vi "monitor_log_queue.vi"(6 "occurrence":refnum<k4>, 11 "File Log Provider in":refnum<data-value>) -> ()   [LabVIEW 2019, in "File Log Provider.lvclass"]
uses:
  File Log Provider.lvclass
  File Log Provider.lvclass/File Log Provider.ctl
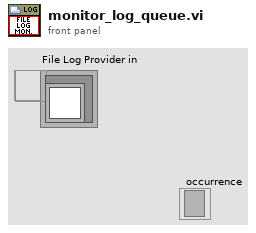
[diagram p1: front panel]
types:
  T1 = enum16{"open", "replace", "create", "open or create", "replace or create", "replace or create with confirmation"}
  T2 = typedef "Queue Log Provider.lvclass/log_message.ctl" = cluster{"Time Stamp":timestamp, "level":T3, "context":string, "message":string}
  T3 = typedef "Utility API.lvlib/Log Service.lvclass/level.ctl" = u16
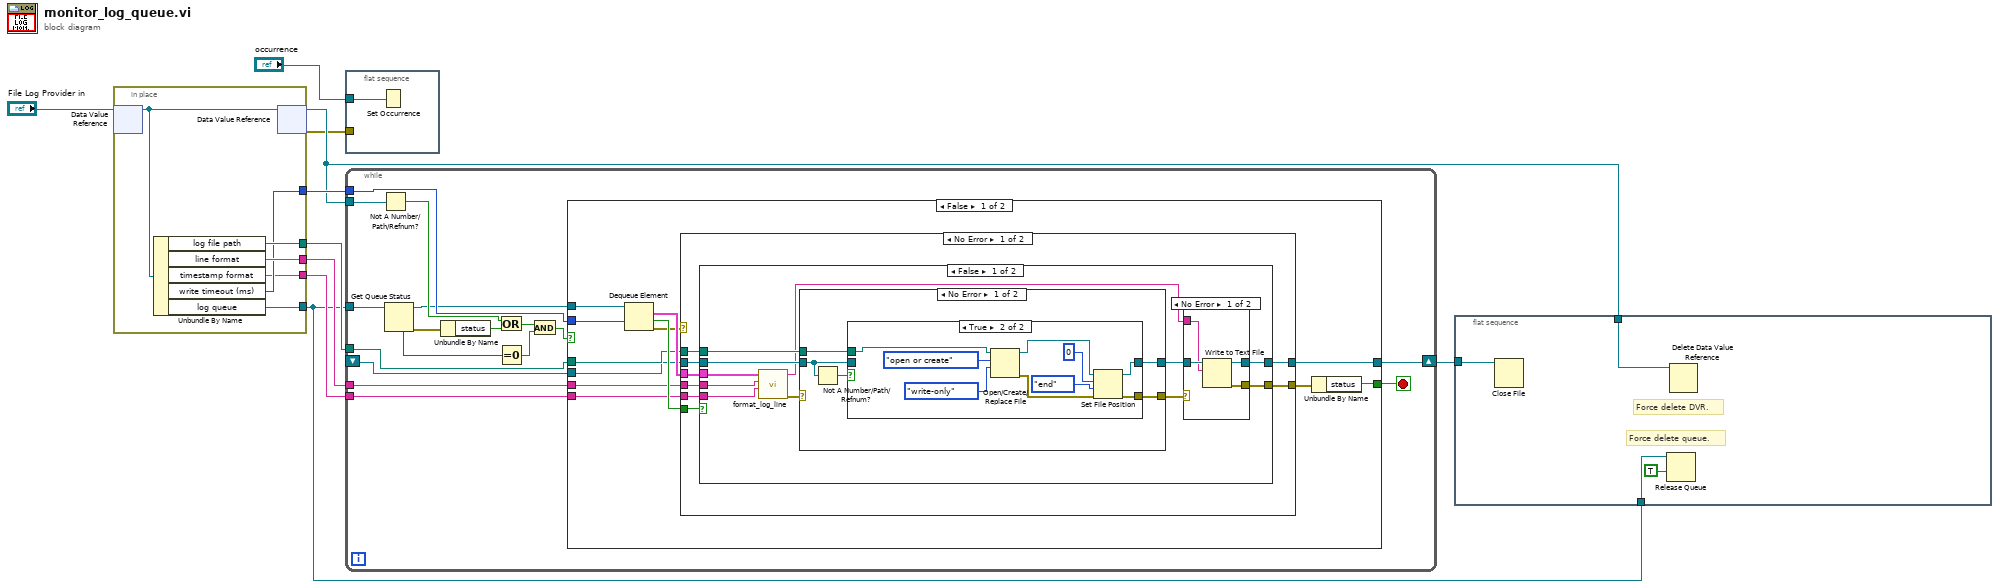
[diagram p0: block diagram]
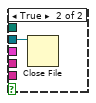
[diagram p5: hidden frame]
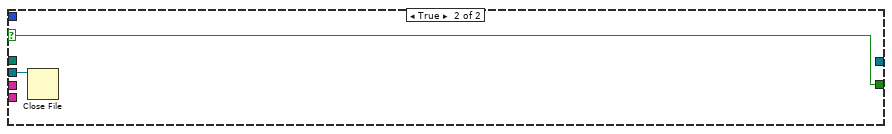
[diagram p7: hidden frame]
diagram:
  n1 = in-place {
    in-place-border: [w15] -> w8
    in-place-border: [w14] -> w7
    in-place-border: [w13] -> w9
    in-place-border: [w12] -> w3
    in-place-border: [w11] -> w6
    n2 = in-place-dvr #1("File Log Provider in") -> (w16:refnum<class "File Log Provider.lvclass">)  [unwired: 1 out]
    n3 = Unbundle By Name(w16) -> ("log file path"=w15:path, "line format"=w14:string, "timestamp format"=w11:string, "write timeout (ms)"=w13:i32, "log queue"=w12:refnum<queue>)
    n4 = in-place-dvr #1(w16) -> (w4:refnum<data-value>, w1:errorcluster)
  }
  n5 = flat-sequence {
    tunnel: "occurrence" -> [w17]
    tunnel: w1 -> [_]
    frame #0 {
      n6 = Set Occurrence(w17) -> ()
    }
  }
  n7 = while {
    tunnel: w4 -> [w34]
    tunnel: w3 -> [w18]
    tunnel: w9 -> [w32]
    tunnel: w8 -> [w31]
    tunnel: w7 -> [w30]
    tunnel: w6 -> [w29]
    shift-right: [w27] -> w5
    shift-left: _ -> [w28]
    stop <- w33 stop-if-true
    n8 = Not A Number/Path/Refnum?(number/path/refnum=w34) -> (NaN/Path/Refnum?=w25:bool)
    n9 = Get Queue Status(queue=w18) -> (queue out=w19:refnum<queue>, error out=w26:errorcluster, # elements in queue=w20:i32)  [unwired: 2 in, 5 out]
    n10 = Unbundle By Name(w26) -> ("status"=w24:bool)
    n11 = Or(x=w25, y=w24) -> (x .or. y?=w23:bool)
    n12 = Equal To 0?(x=w20) -> (x = 0?=w21:bool)
    n13 = And(x=w23, y=w21) -> (x .and. y?=w22:bool)
    n14 = case shown="False" w22 {
      selector: w22 -> [_ w92]
      tunnel: [w44 w92] -> w33
      tunnel: w19 -> [w46 _]
      tunnel: w32 -> [w45 _]
      tunnel: w31 -> [w41 _]
      tunnel: w30 -> [w40 _]
      tunnel: w29 -> [w39 _]
      tunnel: w28 -> [w38 w91]
      tunnel: [w37 _] -> w27
      frame False {
        n15 = Dequeue Element(queue=w46, timeout in ms (-1)=w45) -> (element=w42:T2, timed out?=w43:bool, error out=w36:errorcluster)  [unwired: 1 in, 1 out]
        n16 = case shown="No Error" w36 {
          selector: w36 -> [_ w89]
          tunnel: w43 -> [w54 _]
          tunnel: w42 -> [w53 _]
          tunnel: w41 -> [w52 _]
          tunnel: w40 -> [w51 _]
          tunnel: w39 -> [w50 _]
          tunnel: w38 -> [w49 w90]
          tunnel: [w48 w90] -> w37
          tunnel: [w47 w89] -> w35
          frame No Error {
            n17 = case shown="False" w54 {
              tunnel: w53 -> [w64 _]
              tunnel: w52 -> [w65 _]
              tunnel: w51 -> [w63 _]
              tunnel: w50 -> [w62 _]
              tunnel: w49 -> [w60 w88]
              tunnel: [w57 _] -> w48
              tunnel: [w55 _] -> w47
              frame False {
                n18 = call "format_log_line.vi"("timestamp format"=w62, "line format"=w63, "message"=w64) -> ("error out"=w61:errorcluster, "formatted log line"=w56:string)  [unwired: 7 in]
                n19 = case shown="No Error" w61 {
                  selector: w61 -> [_ w86]
                  tunnel: w65 -> [w75 _]
                  tunnel: [w73 w86] -> w59
                  tunnel: [w72 w87] -> w58
                  tunnel: w60 -> [w71 w87]
                  frame No Error {
                    n20 = Not A Number/Path/Refnum?(number/path/refnum=w71) -> (NaN/Path/Refnum?=w74:bool)
                    n21 = case shown="True" w74 {
                      tunnel: w75 -> [_ w85]
                      tunnel: [w76 w81] -> w72
                      tunnel: [_ w79] -> w73
                      tunnel: w71 -> [w76 _]
                      frame False {
                      }
                      frame True {
                        n22 = Open/Create/Replace File(file path (use dialog)=w85, operation (0:open)=T1."open or create", access (0:read/write)=enum16{"read/write", "read-only", "write-only"}."write-only") -> (refnum out=w82:refnum<file>, error out=w80:errorcluster)  [unwired: 3 in, 1 out]
                        n23 = Set File Position(offset (in bytes) (0)=i64 0, refnum=w82, from (0:start)=enum16{"start", "end", "current"}."end", error in=w80) -> (refnum out=w81:refnum<file>, error out=w79:errorcluster)
                      }
                    }
                  }
                  frame Error {
                  }
                }
                n24 = case shown="No Error" w59 {
                  tunnel: w58 -> [w69 w70]
                  tunnel: [w67 w70] -> w57
                  tunnel: w56 -> [w68 _]
                  tunnel: [w66 _] -> w55
                  frame No Error {
                    n25 = Write to Text File(file (use dialog)=w69, text=w68) -> (refnum out=w67:refnum<file>, error out=w66:errorcluster)  [unwired: 2 in, 1 out]
                  }
                  frame Error {
                  }
                }
              }
              frame True {
                n26 = Close File(refnum=w88) -> ()  [unwired: 1 in, 2 out]
              }
            }
          }
          frame Error {
          }
        }
        n27 = Unbundle By Name(w35) -> ("status"=w44:bool)
      }
      frame True {
        n28 = Close File(refnum=w91) -> ()  [unwired: 1 in, 2 out]
      }
    }
  }
  n29 = flat-sequence {
    tunnel: w5 -> [w93]
    tunnel: w4 -> [w96]
    tunnel: w3 -> [w95]
    frame #0 {
      # "Force delete queue."
      # "Force delete DVR."
      n30 = Close File(refnum=w93) -> ()  [unwired: 1 in, 2 out]
      n31 = Release Queue(queue=w95, force destroy? (F)=TRUE) -> ()  [unwired: 1 in, 3 out]
      n32 = Delete Data Value Reference(data value reference=w96) -> ()  [unwired: 1 in, 2 out]
    }
  }
